vi "Launch Heaters.vi"(8 "error in (no error)":errorcluster, 11 "cRIO-CO2 in":refnum<class "cRIO-CO2.lvclass">=refnum) -> (0 "error out":errorcluster, 3 "cRIO-CO2 out":refnum<class "cRIO-CO2.lvclass">)   [LabVIEW 2015]
uses:
  cRIO-CO2.lvclass
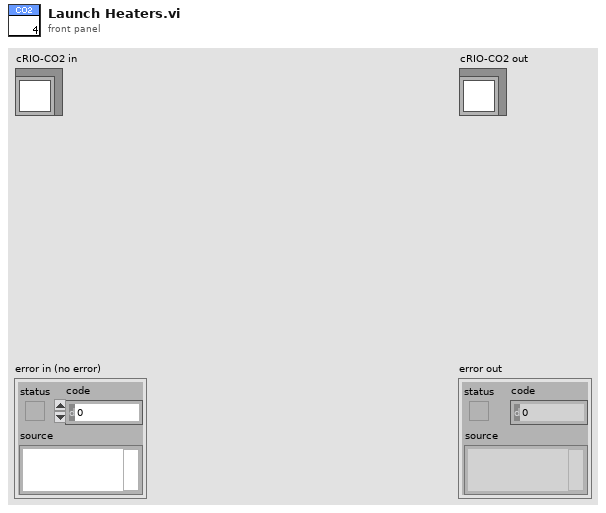
[diagram p1: front panel]
types:
  T1 = cluster{"PID":cluster{"P":dbl, "I":dbl, "D":dbl}, "Setpoint":dbl, "Upper Limit":dbl, "Lower Limit":dbl}
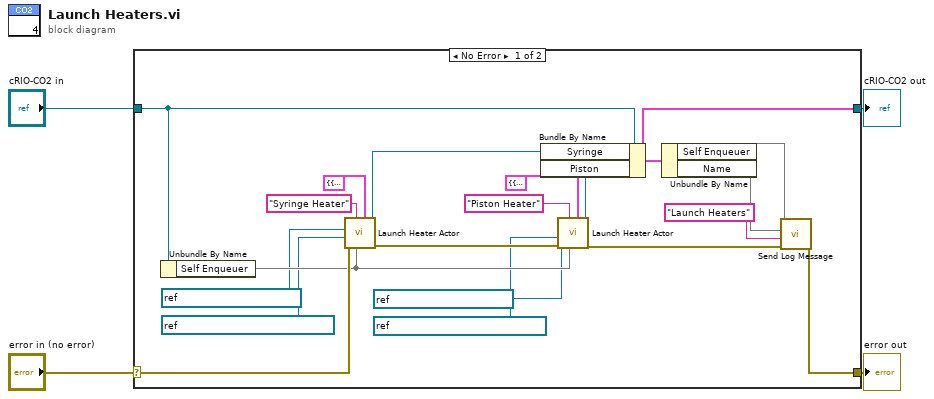
[diagram p0: block diagram]
diagram:
  n1 = case shown="No Error" "error in (no error)" {
    selector: "error in (no error)" -> [w23 w26]
    tunnel: [w15 w26] -> w3
    tunnel: [w20 w25] -> w1
    tunnel: "cRIO-CO2 in" -> [w14 w25]
    frame No Error {
      n2 = Unbundle By Name(w14) -> ("Self Enqueuer"=w13)
      n3 = call "Launch Heater Actor.vi"("PID."=T1 {"PID"={"P"=20.0, "I"=2.0, "D"=10.0}, "Setpoint"=25.0, "Upper Limit"=1000.0, "Lower Limit"=-100.0}, "SHVs"=w13, "Name"="Syringe Heater", "error in (no error)"=w23, 9:refnum<k21> "ni.var.io://10.2.0.20/EtherCAT Master/Device/User-Defined Variables/Syringe Heater Duty Cycle (‰)" ("Heater Duty Cycle SHV"), "Interlock Chain"=refnum<k21> "ni.var.io://10.2.0.20/EtherCAT Master/Device/Mod2/Syringe TC" ("Thermocouple SHV")) -> ("error out"=w22:errorcluster, "Caller-To-Actor Enqueuer"=w24:refnum<class "Message Enqueuer.lvclass">)  [unwired: 4 in]
      n4 = call "Launch Heater Actor.vi"("PID."=T1 {"PID"={"P"=10.0, "I"=1.5, "D"=5.0}, "Setpoint"=25.0, "Upper Limit"=100.0, "Lower Limit"=-20.0}, "SHVs"=w13, "Name"="Piston Heater", "error in (no error)"=w22, 9:refnum<k21> "ni.var.io://10.2.0.20/EtherCAT Master/Device/User-Defined Variables/Piston Heater Duty Cycle (‰)" ("Heater Duty Cycle SHV"), "Interlock Chain"=refnum<k21> "ni.var.io://10.2.0.20/EtherCAT Master/Device/Mod2/Piston TC" ("Thermocouple SHV")) -> ("error out"=w16:errorcluster, "Caller-To-Actor Enqueuer"=w21:refnum<class "Message Enqueuer.lvclass">)  [unwired: 4 in]
      n5 = Bundle By Name(cluster=w14, "Syringe"=w24, "Piston"=w21) -> (w20:cluster{})
      n6 = Unbundle By Name(w20) -> ("Self Enqueuer"=w19, "Name"=w18)
      n7 = call "Send Log Message.vi"("error in (no error)"=w16, "String"="Launch Heaters", "Source Name"=w18, "Message Enqueuer"=w19) -> ("error out"=w15:errorcluster)  [unwired: 6 in, 1 out]
    }
    frame Error {
    }
  }
  "error out" <- w3
  "cRIO-CO2 out" <- w1
